vi "BH Druck  PACE Series Vent.vi"() -> ()   [LabVIEW 2022 SP3]
uses:
  BH Druck PACE Series.lvclass
panel:
  in  "Channel (0: Channel A)":u16(ring) items=["Channel A", "Channel B"]
  out "Vent Status":i32
  in  "VISA resource name":refnum<visa-resource-name>
  # "(c)2020 BH  Druck Ltd.  ALL RIGHTS RESERVED."
  # "This example demonstrates the application of Enable Vent.vi and Vent Status.vi.  \nIt opens the Vent valve and queries the vent process until it finishes."
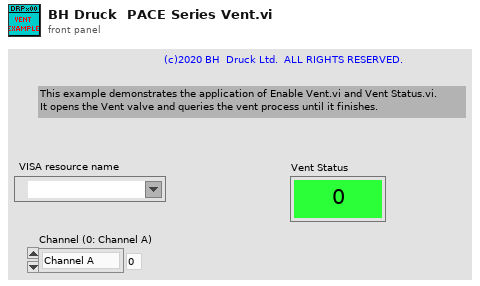
[diagram p1: front panel]
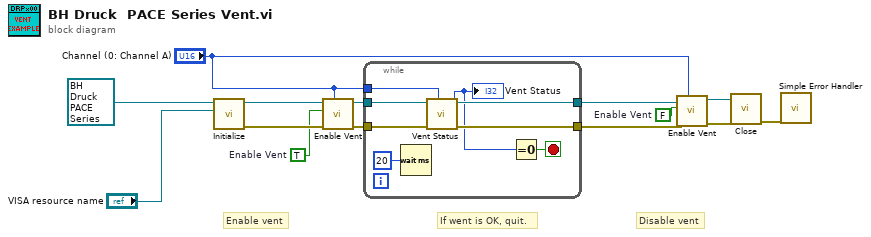
[diagram p0: block diagram]
diagram:
  w3 = FALSE  # Enable Vent
  w4 = TRUE  # Enable Vent
  # "Disable vent"
  # "If went is OK, quit."
  # "Enable vent"
  n1 = call-dynamic "Initialize.vi"("VISA resource name"="VISA resource name", "BH Druck PACE Series in"=refnum<class "BH Druck PACE Series.lvclass"> refnum) -> ("error out"=w13:errorcluster, "BH Druck PACE Series out"=w14:refnum<class "BH Druck PACE Series.lvclass">)  [unwired: 7 in]
  n2 = call-dynamic "Enable Vent.vi"("Channel (0: Channel A)"="Channel (0: Channel A)", "error in (no error)"=w13, "Enable Vent (T: On)"=w4, "BH Druck PACE Series in"=w14) -> ("error out"=w11:errorcluster, "BH Druck PACE Series out"=w12:refnum<class "BH Druck PACE Series.lvclass">)  [unwired: 6 in]
  n3 = while {
    tunnel: "Channel (0: Channel A)" -> [w15]
    tunnel: w12 -> [w22]
    tunnel: [w20] -> w10
    tunnel: w11 -> [w21]
    tunnel: [w19] -> w9
    stop <- w16 stop-if-true
    n4 = Wait (ms)(milliseconds to wait=u32 20) -> ()  [unwired: 1 out]
    n5 = call-dynamic "Vent Status.vi"("Channel (0: Channel A)"=w15, "error in (no error)"=w21, "BH Druck PACE Series in"=w22) -> ("error out"=w19:errorcluster, "Vent Status"=w17:i32, "BH Druck PACE Series out"=w20:refnum<class "BH Druck PACE Series.lvclass">)  [unwired: 6 in]
    "Vent Status" <- w17
    n6 = Equal To 0?(x=w17) -> (x = 0?=w16:bool)
  }
  n7 = call-dynamic "Enable Vent.vi"("Channel (0: Channel A)"="Channel (0: Channel A)", "error in (no error)"=w9, "Enable Vent (T: On)"=w3, "BH Druck PACE Series in"=w10) -> ("error out"=w7:errorcluster, "BH Druck PACE Series out"=w8:refnum<class "BH Druck PACE Series.lvclass">)  [unwired: 6 in]
  n8 = call "Close.vi"("error in (no error)"=w7, "BH Druck PACE Series in"=w8) -> ("error out"=w2:errorcluster)  [unwired: 8 in, 1 out]
  n9 = call <vilib>:"Simple Error Handler.vi"("error in (no error)"=w2) -> ()  [unwired: 4 in, 5 out]
